vi "sv_UFF58 Check Data Valid.vi"   [LabVIEW 2017, in "SoundVib_UFF58.lvlib"]
doc: "Check if the input waveform(s) or spectrum(spectra) is empty. Returns an error if the input is empty"
uses:
  <vilib>/addons/Sound and Vibration/svt_UFF58/SoundVib_UFF58.lvlib
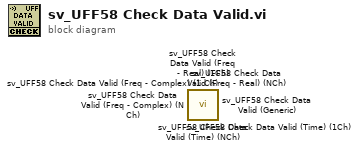
[diagram p0: block diagram]
diagram:
  n1 = call <vilib>:"sv_UFF58 Check Data Valid (Time) (NCh).vi"() -> ()  [unwired: 14 in, 2 out]
  n2 = call <vilib>:"sv_UFF58 Check Data Valid (Freq - Real) (NCh).vi"() -> ()  [unwired: 14 in, 2 out]
  n3 = call <vilib>:"sv_UFF58 Check Data Valid (Freq - Complex) (N Ch).vi"() -> ()  [unwired: 12 in, 4 out]
  n4 = call <vilib>:"sv_UFF58 Check Data Valid (Generic).vi"() -> ()  [unwired: 12 in, 4 out]
  n5 = call <vilib>:"sv_UFF58 Check Data Valid (Freq - Complex) (1 Ch).vi"() -> ()  [unwired: 12 in, 4 out]
  n6 = call <vilib>:"sv_UFF58 Check Data Valid (Freq - Real) (1Ch).vi"() -> ()  [unwired: 13 in, 3 out]
  n7 = call <vilib>:"sv_UFF58 Check Data Valid (Time) (1Ch).vi"() -> ()  [unwired: 14 in, 2 out]
